vi "Patty test.vi"() -> ()   [LabVIEW 2016]
uses:
  Actuator/Controls/Command cluster.ctl
  Actuator/Controls/Command list.ctl
  General/Controls/data modes.ctl
panel:
  out "Load":dbl(graph)
  out "P v L":cluster{dbl[], dbl[]}(graph)
  out "L v T":cluster{dbl[], dbl[]}(graph)
  out "P v T":cluster{dbl[], dbl[]}(graph)
  out "Position":dbl(graph)
  in  "Abort":bool
  in  "VISA resource name":refnum<visa-resource-name>="COM4"
  out "Device Information":string
  out "Testing?":bool
  in  "Test":bool
  out "Force (mN)":dbl
  in  "Speed (mm/s)":dbl=3.0 min=0.1 max=25.0 step=0.1
  out "Position (mm)":dbl
  out "x-y":u32
  out "error out":errorcluster={"status"=FALSE, "code"=1073676294, "source"="VISA Read in SMAC Parameters.vi->SMAC LabVIEW Toolkit_v1.vi"}
  in  "Set point":dbl
  in  "stop":bool
  in  "error in (no error)":errorcluster
  # "Use 'W' and 'S' keys to move the actuator up and down"
  # "- Filename and folder save (metadata + user field)\n- Calibration for load cell"
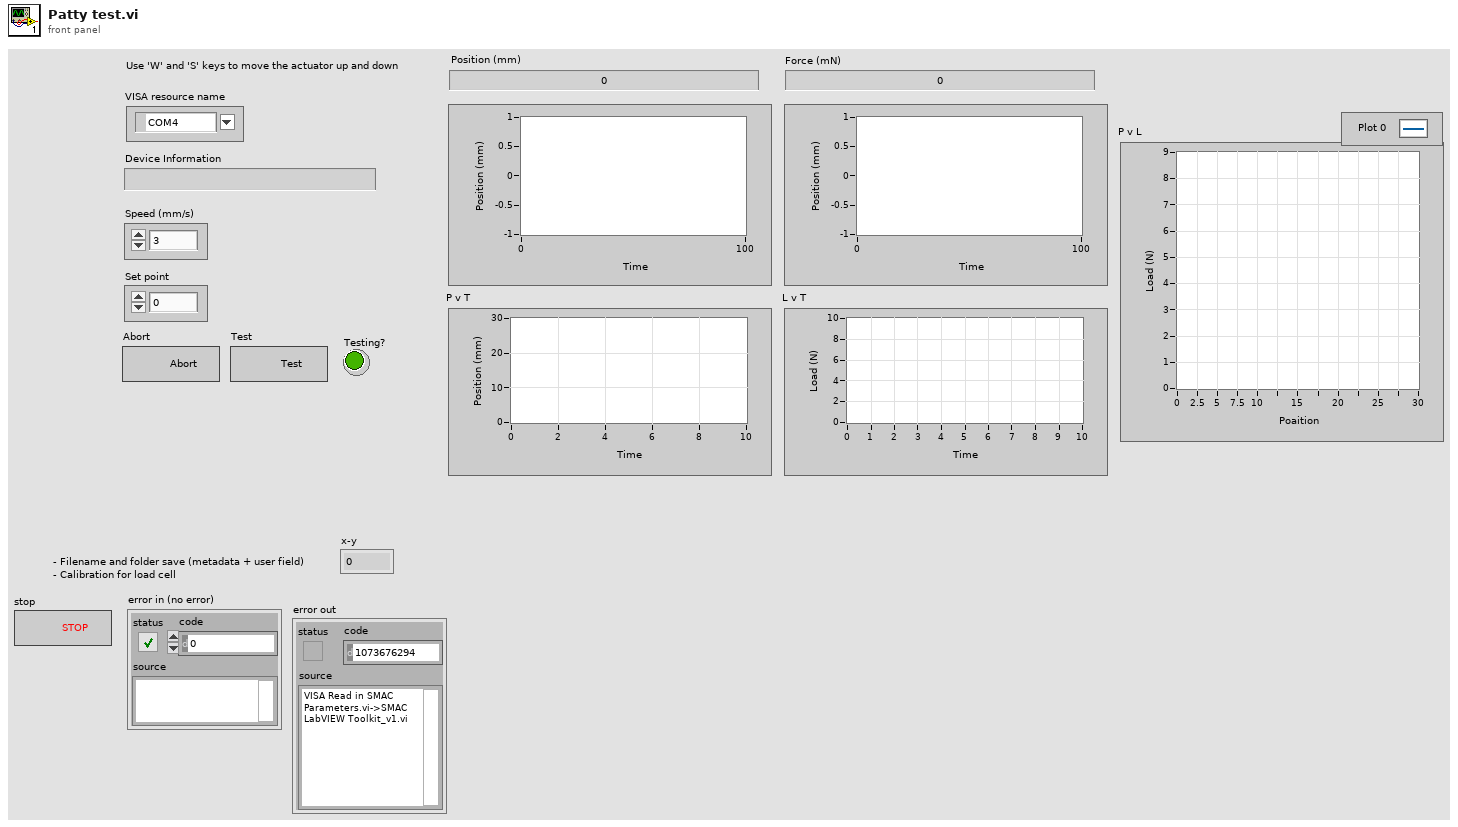
[diagram p1: front panel]
types:
  T1 = typedef "data modes.ctl" = enum16{"Initalise", "Status", "Process", "Add load", "Add position"}
  T2 = typedef "Command cluster.ctl" = cluster{"Command":T3, "data":variant}
  T3 = typedef "Command list.ctl" = enum16{"", "£nabort", "getaxisno", "£getserialno", "£nidentify", "&&£setnlimit", "&£nm", "&£snv", "&£speed", "£np", "£ncal"}
  T4 = cluster{"seconds since 1Jan1904":timestamp, "data":dbl}[]
  T5 = cluster{"seconds since 1Jan1904":timestamp, "data":dbl}
  T6 = enum16{"open", "replace", "create", "open or create", "replace or create", "replace or create with confirmation"}
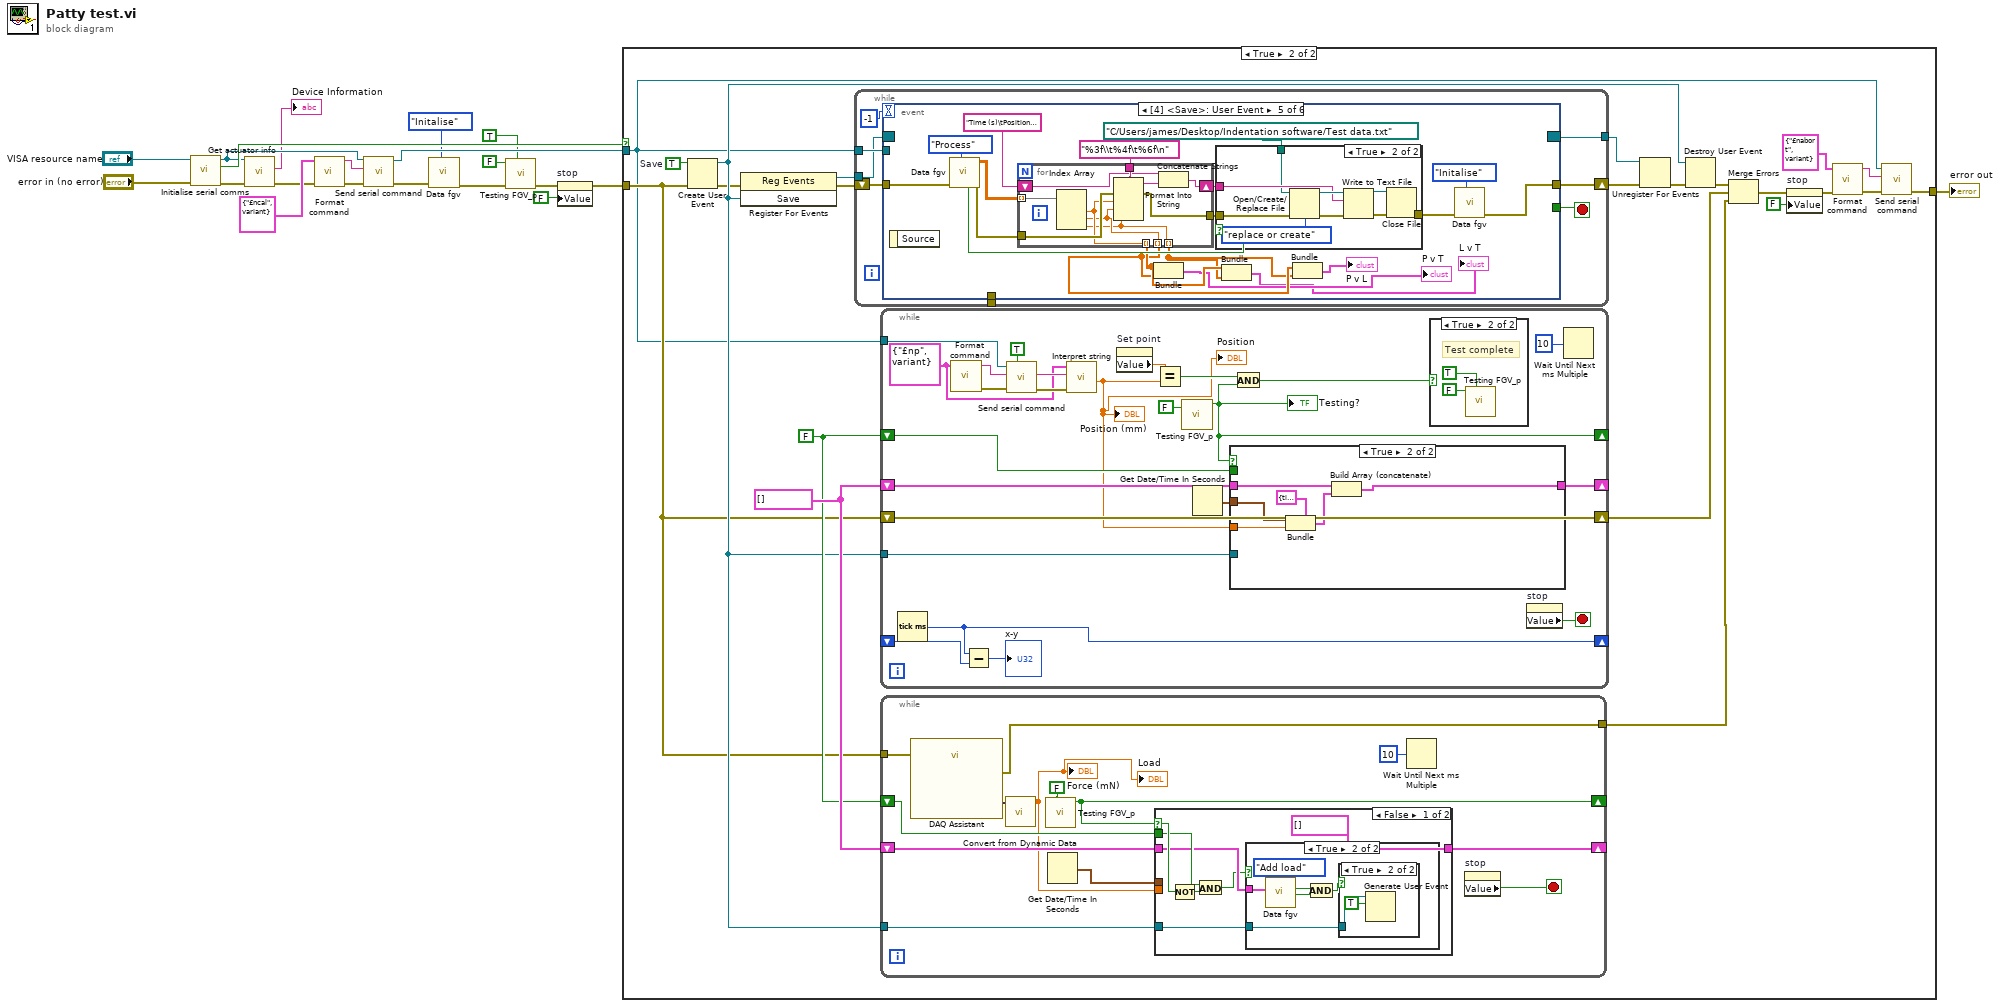
[diagram p0: block diagram]
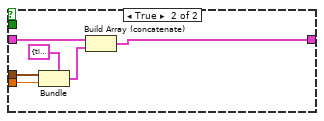
[diagram p5: hidden frame]
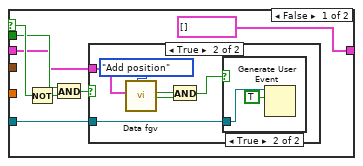
[diagram p6: hidden frame]
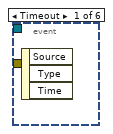
[diagram p10: hidden frame]
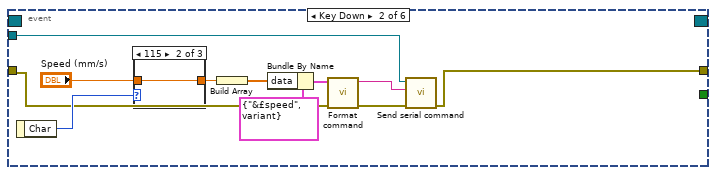
[diagram p11: hidden frame]
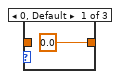
[diagram p12: hidden frame]
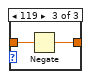
[diagram p13: hidden frame]
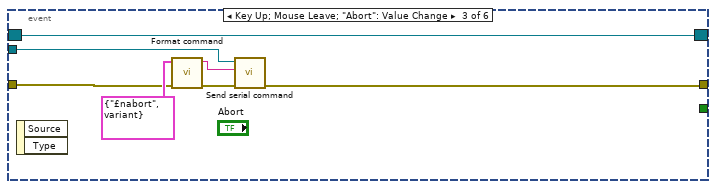
[diagram p14: hidden frame]
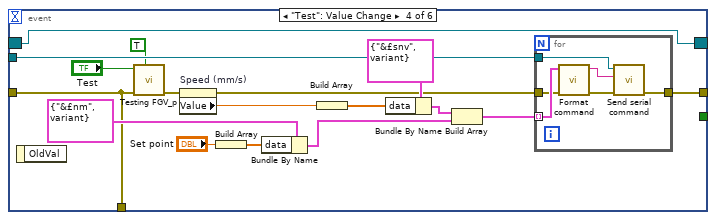
[diagram p15: hidden frame]
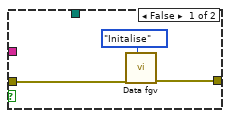
[diagram p16: hidden frame]
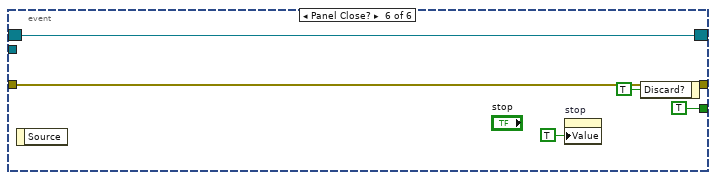
[diagram p17: hidden frame]
diagram:
  n1 = call "Initialise serial comms.vi"("error in (no error)"="error in (no error)", "VISA Refnum in"="VISA resource name") -> ("error out"=w20:errorcluster, "Connected?"=w14:bool, "VISA Refnum out"=w13:refnum<visa-resource-name>)  [unwired: 7 in]
  n2 = call "Get actuator info.vi"("error in (no error)"=w20, "VISA Refnum in"=w13) -> ("error out"=w17:errorcluster, "String"=→"Device Information":string)  [unwired: 7 in, 1 out]
  n3 = call "Format command.vi"("error in (no error)"=w17, "Cluster"=T2 {"Command"=enum."£ncal", "data"=variant}) -> ("error out"=w16:errorcluster, "String"=w15:string)  [unwired: 8 in]
  n4 = call "Send serial command.vi"("error IO"=w16, "Send string"=w15, "VISA resource name out"=w13) -> ("error out"=w8:errorcluster, "VISA Out"=w12:refnum<visa-resource-name>)  [unwired: 6 in, 1 out]
  n5 = call "Data fgv.vi"("Modes"=data_modes."Initalise", "error in (no error)"=w8) -> ("error out"=w7:errorcluster)  [unwired: 5 in, 4 out]
  n6 = call "Testing FGV_p.vi"("Set"=TRUE, "error in (no error)"=w7, "Value"=FALSE) -> ("error out"=w6:errorcluster)  [unwired: 7 in, 1 out]
  n7 = property on="stop" class="Bool (strict)"(error in=w6, "Value"=FALSE ("stop")) -> (error out=w5:errorcluster)  [unwired: 1 in, 1 out]
  n8 = case shown="True" w14 {
    tunnel: w12 -> [_ w22]
    tunnel: w5 -> [w21 w29]
    tunnel: [w21 w23] -> w3
    frame False {
    }
    frame True {
      w41 = TRUE  # Save
      w43 = T4 [] ("Data")
      w42 = FALSE ("Testing?")
      n9 = Create User Event(user event datatype=w41, error in=w29) -> (user event=w37:refnum<user-event>, error out=w36:errorcluster)
      n10 = register-events(error in=w36, w37) -> (reference out=w40:refnum<event-registration>, error out=w35:errorcluster)  [unwired: 1 in]
      n11 = while {
        tunnel: w22 -> [w131]
        tunnel: [w129] -> _
        tunnel: w40 -> [w128]
        tunnel: [w127] -> w39
        shift-right: [w125] -> w34
        shift-left: w35 -> [w130]
        stop <- w126 stop-if-true
        n12 = event shown="[4] <Save>: User Event" {
          selector: w128 -> [_ _ w148 w155 _ w222]
          dyn-events: [_ _ w148 w155 _ w222] -> w127
          timeout: -1 -> [_ _ _ _ _ _]
          tunnel: w131 -> [_ w138 w152 w170 _ _]
          tunnel: w130 -> [_ w134 w150 w159 w196 w221]
          tunnel: [_ _ _ w159 _ _] -> w129
          tunnel: [_ _ _ _ _ TRUE] -> w126
          tunnel: [_ w133 w149 w156 w184 w221] -> w125
          event Timeout {
            n13 = event-data() -> ()  [unwired: 1 in, 3 out]
          }
          event Key Down {
            n14 = event-data() -> ("Char"=w137:i16)  [unwired: 1 in]
            n15 = case shown="115" w137 {
              tunnel: [0.0 w145 w147] -> w142
              tunnel: "Speed (mm/s)" -> [_ w145 w146]
              frame 0, Default {
              }
              frame 115 {
              }
              frame 119 {
                n16 = Negate(x=w146) -> (-x=w147:dbl)
              }
            }
            n17 = Build Array(w142) -> (w141:dbl[])
            n18 = Bundle By Name(cluster=T2 {"Command"=enum."&£speed", "data"=variant} ("Cluster"), "data"=w141) -> (w140:T2)
            n19 = call "Format command.vi"("error in (no error)"=w134, "Cluster"=w140) -> ("error out"=w135:errorcluster, "String"=w139:string)  [unwired: 8 in]
            n20 = call "Send serial command.vi"("error IO"=w135, "Send string"=w139, "VISA resource name out"=w138) -> ("error out"=w133:errorcluster)  [unwired: 6 in, 2 out]
          }
          event Key Up; Mouse Leave; "Abort": Value Change {
            n21 = event-data() -> ()  [unwired: 1 in, 2 out]
            n22 = call "Format command.vi"("error in (no error)"=w150, "Cluster"=T2 {"Command"=enum."£nabort", "data"=variant} ("Cluster 2")) -> ("error out"=w153:errorcluster, "String"=w154:string)  [unwired: 8 in]
            n23 = call "Send serial command.vi"("error IO"=w153, "Send string"=w154, "VISA resource name out"=w152) -> ("error out"=w149:errorcluster)  [unwired: 6 in, 2 out]
          }
          event "Test": Value Change {
            n24 = event-data() -> ()  [unwired: 1 in, 1 out]
            n25 = call "Testing FGV_p.vi"("Set"=TRUE, "error in (no error)"=w159, "Value"="Test") -> ("error out"=w158:errorcluster)  [unwired: 7 in, 1 out]
            n26 = property on="Speed (mm/s)" class="DigNum (strict)"(error in=w158) -> (error out=w157:errorcluster, "Value"=w162:dbl)  [unwired: 1 in, 1 out]
            n27 = Build Array("Set point") -> (w165:dbl[])
            n28 = Bundle By Name(cluster=T2 {"Command"=enum."&£nm", "data"=variant} ("Cluster"), "data"=w165) -> (w164:T2)
            n29 = Build Array(w162) -> (w163:dbl[])
            n30 = Bundle By Name(cluster=T2 {"Command"=enum."&£snv", "data"=variant} ("Cluster"), "data"=w163) -> (w167:T2)
            n31 = Build Array(w167, w164) -> (w169:T2[])
            n32 = for {
              tunnel: w170 -> [w176]
              tunnel: w169 -> [w174] mode=indexing
              tunnel: w157 -> [w173]
              tunnel: [w172] -> w156
              n33 = call "Format command.vi"("error in (no error)"=w173, "Cluster"=w174) -> ("error out"=w177:errorcluster, "String"=w175:string)  [unwired: 8 in]
              n34 = call "Send serial command.vi"("error IO"=w177, "Send string"=w175, "VISA resource name out"=w176) -> ("error out"=w172:errorcluster)  [unwired: 6 in, 2 out]
            }
          }
          event User Event {
            n35 = event-data() -> ()  [unwired: 1 in, 1 out]
            n36 = call "Data fgv.vi"("Modes"=data_modes."Process", "error in (no error)"=w196) -> ("error out"=w189:errorcluster, "appended array"=w190:dbl[][], "Data"=w188:bool)  [unwired: 5 in, 2 out]
            n37 = for {
              tunnel: "%3f\\t%4f\t%6f\n" ("format string") -> [w218]
              shift-right: [w215] -> w192
              shift-left: "Time (s)\tPosition (mm)\tLoad (N)\n" ("format string") -> [w216]
              tunnel: w190 -> [w214] mode=indexing
              tunnel: w189 -> [w213]
              tunnel: [w212] -> w191
              tunnel: [w211] -> w183 mode=indexing
              tunnel: [w210] -> w182 mode=indexing
              tunnel: [w209] -> w181 mode=indexing
              n38 = Index Array(array=w214) -> (element #1=w211:dbl, element #2=w210:dbl, element #3=w209:dbl)  [unwired: 3 in]
              n39 = Format Into String(format string=w218, error in=w213, w211, w210, w209) -> (resulting string=w217:string, error out=w212:errorcluster)  [unwired: 1 in]
              n40 = Concatenate Strings(w216, w217) -> (w215:string)
            }
            n41 = Bundle(w183, w182) -> (→"P v T":cluster{dbl[], dbl[]})  [unwired: 1 in]
            n42 = case shown="True" w188 {
              tunnel: path "C:/Users/james/Desktop/Indentation software/Test data.txt" ("file path (use dialog)") -> [_ w200]
              tunnel: w192 -> [_ w204]
              tunnel: w191 -> [w199 w202]
              tunnel: [w197 w201] -> w186
              frame False {
                n43 = call "Data fgv.vi"("Modes"=data_modes."Initalise", "error in (no error)"=w199) -> ("error out"=w197:errorcluster)  [unwired: 5 in, 4 out]
              }
              frame True {
                n44 = Open/Create/Replace File(file path (use dialog)=w200, error in=w202, operation (0:open)=T6."replace or create") -> (refnum out=w205:refnum<file>, error out=w203:errorcluster)  [unwired: 3 in, 1 out]
                n45 = Write to Text File(file (use dialog)=w205, text=w204, error in=w203) -> (refnum out=w208:refnum<file>, error out=w207:errorcluster)  [unwired: 1 in, 1 out]
                n46 = Close File(refnum=w208, error in=w207) -> (error out=w201:errorcluster)  [unwired: 1 out]
              }
            }
            n47 = Bundle(w183, w181) -> (→"L v T":cluster{dbl[], dbl[]})  [unwired: 1 in]
            n48 = Bundle(w182, w181) -> (→"P v L":cluster{dbl[], dbl[]})  [unwired: 1 in]
            n49 = call "Data fgv.vi"("Modes"=data_modes."Initalise", "error in (no error)"=w186) -> ("error out"=w184:errorcluster)  [unwired: 5 in, 4 out]
          }
          event Panel Close? {
            n50 = event-data() -> ()  [unwired: 1 in, 1 out]
            n51 = property on="stop" class="Bool (strict)"("Value"=TRUE ("stop")) -> ()  [unwired: 2 in, 2 out]
            n52 = event-data("Discard?"=TRUE) -> ()  [unwired: 1 in, 1 out]
          }
        }
      }
      n53 = while {
        tunnel: w22 -> [w99]
        shift-right: [w97] -> _
        shift-left: _ -> [w96]
        shift-right: [w85] -> _
        shift-left: w43 -> [w89]
        shift-right: [w86] -> _
        shift-left: w42 -> [w87]
        tunnel: w37 -> [w84]
        shift-right: [w83] -> w30
        shift-left: w29 -> [w83]
        stop <- w82 stop-if-true
        w79 = T2 {"Command"=enum."£np", "data"=variant} ("Cluster")
        n54 = Tick Count (ms)() -> (millisecond timer value=w97:u32)
        n55 = call "Format command.vi"("Cluster"=w79) -> ("error out"=w81:errorcluster, "String"=w100:string)  [unwired: 9 in]
        n56 = Subtract(x=w97, y=w96) -> (x-y=→"x-y":u32)
        n57 = call "Send serial command.vi"("Read?"=TRUE, "error IO"=w81, "Send string"=w100, "VISA resource name out"=w99) -> ("error out"=w80:errorcluster, "read string"=w94:string)  [unwired: 5 in, 1 out]
        n58 = call "Interpret string.vi"("error in (no error)"=w80, "String"=w94, "Cluster"=w79) -> ("Numeric 2"=w78:dbl)  [unwired: 5 in, 3 out]
        "Position (mm)" <- w78
        "Position" <- w78
        n59 = property on="Set point" class="DigNum (strict)"() -> ("Value"=w93:dbl)  [unwired: 2 in, 2 out]
        n60 = Equal?(x=w93, y=w78) -> (x = y?=w92:bool)
        n61 = call "Testing FGV_p.vi"("Set"=FALSE) -> ("Testing?"=w86:bool)  [unwired: 9 in, 1 out]
        "Testing?" <- w86
        n62 = Get Date/Time In Seconds() -> (seconds since 1Jan1904=w88:timestamp)
        n63 = case shown="True" w86 {
          selector: w86 -> [w107 _]
          tunnel: w88 -> [_ w121]
          tunnel: w78 -> [_ w120]
          tunnel: w87 -> [w105 _]
          tunnel: w89 -> [w104 w119]
          tunnel: [T4 [] w117] -> w85
          tunnel: w84 -> [w102 _]
          frame False {
            n64 = Not(x=w107) -> (.not. x?=w106:bool)
            n65 = And(x=w105, y=w106) -> (x .and. y?=w103:bool)
            n66 = case shown="True" w103 {
              tunnel: w104 -> [_ w113]
              tunnel: w102 -> [_ w109]
              frame False {
              }
              frame True {
                n67 = call "Data fgv.vi"("Modes"=data_modes."Add position", "Data"=w113) -> ("Load?"=w111:bool, "Position?"=w112:bool)  [unwired: 5 in, 3 out]
                n68 = And(x=w112, y=w111) -> (x .and. y?=w110:bool)
                n69 = case shown="True" w110 {
                  tunnel: w109 -> [_ w116]
                  frame False {
                  }
                  frame True {
                    n70 = Generate User Event(user event=w116, event data cluster=TRUE ("event data")) -> ()  [unwired: 2 in, 2 out]
                  }
                }
              }
            }
          }
          frame True {
            n71 = Bundle(cluster=T5 {"seconds since 1Jan1904"=timestamp(0 s since 1904-01-01), "data"=0.0} ("element"), "seconds since 1Jan1904"=w121, "data"=w120) -> (w118:T5)
            n72 = Build Array (concatenate)(w119, w118) -> (w117:T4)
          }
        }
        n73 = And(x=w92, y=w86) -> (x .and. y?=w90:bool)
        n74 = case shown="True" w90 {
          frame False {
          }
          frame True {
            # "Test complete"
            n75 = call "Testing FGV_p.vi"("Set"=TRUE, "Value"=FALSE) -> ()  [unwired: 8 in, 2 out]
          }
        }
        n76 = property on="stop" class="Bool (strict)"() -> ("Value"=w82:bool)  [unwired: 2 in, 2 out]
        n77 = Wait Until Next ms Multiple(millisecond multiple=u32 10) -> ()  [unwired: 1 out]
      }
      n78 = while {
        shift-right: [w52] -> _
        shift-left: w42 -> [w51]
        shift-right: [w49] -> _
        shift-left: w43 -> [w50]
        tunnel: w37 -> [w48]
        tunnel: w29 -> [w47]
        tunnel: [w46] -> w28
        stop <- w45 stop-if-true
        n79 = call "DAQ Assistant"("error in"=w47) -> ("data"=w56:dynamicdata, "error out"=w46:errorcluster)  [unwired: 16 in, 1 out]
        n80 = call "Convert from Dynamic Data"("Dynamic Data Type"=w56) -> ("Scalar"=w44:dbl)  [unwired: 3 in]
        "Force (mN)" <- w44
        "Load" <- w44
        n81 = call "Testing FGV_p.vi"("Set"=FALSE) -> ("Testing?"=w52:bool)  [unwired: 9 in, 1 out]
        n82 = Get Date/Time In Seconds() -> (seconds since 1Jan1904=w54:timestamp)
        n83 = case shown="False" w52 {
          selector: w52 -> [w62 _]
          tunnel: w54 -> [_ w76]
          tunnel: w44 -> [_ w75]
          tunnel: w51 -> [w60 _]
          tunnel: w50 -> [w59 w74]
          tunnel: [T4 [] w72] -> w49
          tunnel: w48 -> [w57 _]
          frame False {
            n84 = Not(x=w62) -> (.not. x?=w61:bool)
            n85 = And(x=w60, y=w61) -> (x .and. y?=w58:bool)
            n86 = case shown="True" w58 {
              tunnel: w59 -> [_ w68]
              tunnel: w57 -> [_ w64]
              frame False {
              }
              frame True {
                n87 = call "Data fgv.vi"("Modes"=data_modes."Add load", "Data"=w68) -> ("Load?"=w66:bool, "Position?"=w67:bool)  [unwired: 5 in, 3 out]
                n88 = And(x=w67, y=w66) -> (x .and. y?=w65:bool)
                n89 = case shown="True" w65 {
                  tunnel: w64 -> [_ w71]
                  frame False {
                  }
                  frame True {
                    n90 = Generate User Event(user event=w71, event data cluster=TRUE ("event data")) -> ()  [unwired: 2 in, 2 out]
                  }
                }
              }
            }
          }
          frame True {
            n91 = Bundle(cluster=T5 {"seconds since 1Jan1904"=timestamp(0 s since 1904-01-01), "data"=0.0} ("element"), "seconds since 1Jan1904"=w76, "data"=w75) -> (w73:T5)
            n92 = Build Array (concatenate)(w74, w73) -> (w72:T4)
          }
        }
        n93 = Wait Until Next ms Multiple(millisecond multiple=u32 10) -> ()  [unwired: 1 out]
        n94 = property on="stop" class="Bool (strict)"() -> ("Value"=w45:bool)  [unwired: 2 in, 2 out]
      }
      n95 = Unregister For Events(event registration refnum=w39, error in=w34) -> (error out=w38:errorcluster)
      n96 = Destroy User Event(user event=w37, error in=w38) -> (error out=w33:errorcluster)
      n97 = Merge Errors(w33, w30, w28) -> (w32:errorcluster)
      n98 = property on="stop" class="Bool (strict)"(error in=w32, "Value"=FALSE ("stop")) -> (error out=w24:errorcluster)  [unwired: 1 in, 1 out]
      n99 = call "Format command.vi"("error in (no error)"=w24, "Cluster"=T2 {"Command"=enum."£nabort", "data"=variant} ("Cluster 2")) -> ("error out"=w25:errorcluster, "String"=w26:string)  [unwired: 8 in]
      n100 = call "Send serial command.vi"("error IO"=w25, "Send string"=w26, "VISA resource name out"=w22) -> ("error out"=w23:errorcluster)  [unwired: 6 in, 2 out]
    }
  }
  "error out" <- w3
